vi "Cryotel Status.vi"(8 "Number of reads":i32, 11 "VISA Resource (write)":refnum<visa-resource-name>="COM1") -> (0 "Array 2":dbl[](array[numeric]), 3 "read string array":string[](array[string]))   [LabVIEW 2020]
uses:
  <vilib>/Analysis/baseanly.llb/Mean (DBL).vi
  <vilib>/Analysis/NI_AALBase.lvlib
panel:
  out "Array":string[](array[string])
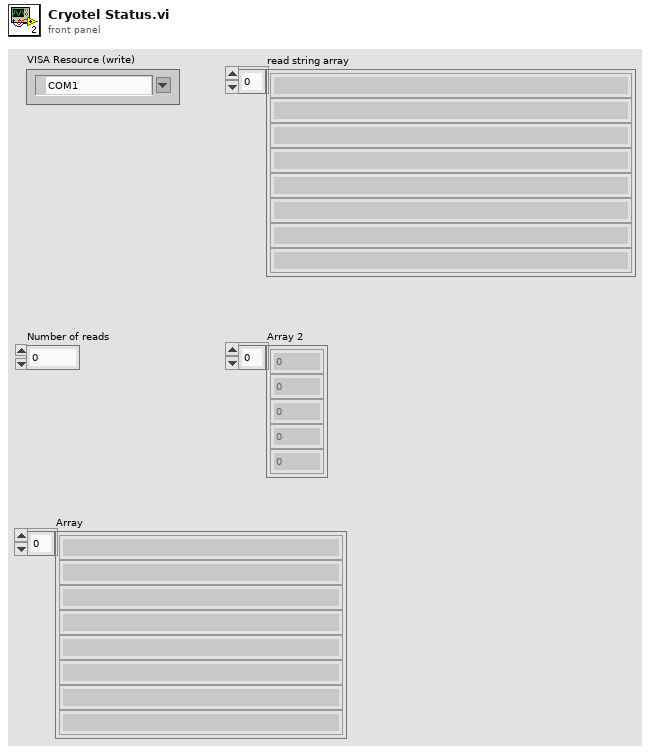
[diagram p1: front panel]
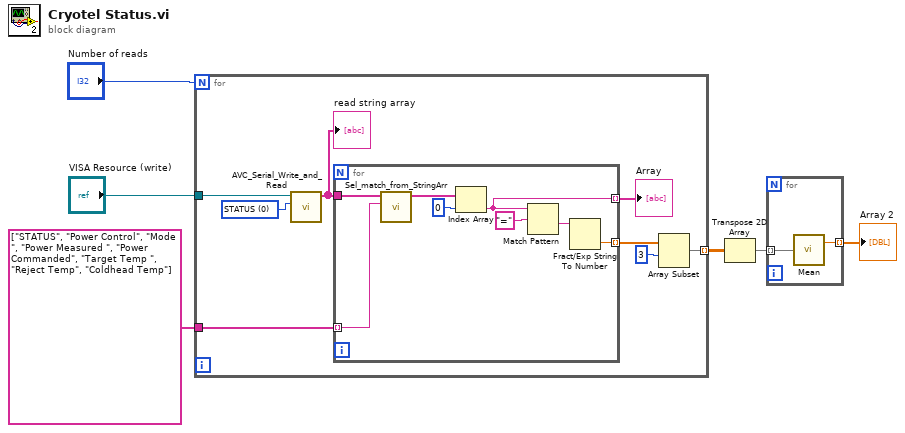
[diagram p0: block diagram]
diagram:
  n1 = for {
    N: "Number of reads" -> [_]
    tunnel: [w11] -> w2 mode=indexing
    tunnel: string[] ["STATUS", "Power Control", "Mode  ", "Power Measured ", "Power Commanded", "Target Temp ", "Reject Temp", "Coldhead Temp"] -> [w9]
    tunnel: "VISA Resource (write)" -> [w8]
    w7 = u16 0 items=["STATUS", "COOLER", "E", "ERROR", "KD", "KI", "KP", "LOGIN", "LOGOUT", "MODE", "P", "PWOUT", "SENSOR", "TC", "TEMP RJ", "TTARGET", "VERSION"] ("Command")
    n2 = call "AVC_Serial_Write_and_Read.vi"("Command"=w7, "VISA Resource (write)"=w8) -> ("read string array"=w10:string[])  [unwired: 8 in, 1 out]
    "read string array" <- w10
    n3 = for {
      tunnel: w10 -> [w22]
      tunnel: [w18] -> w14 mode=indexing
      tunnel: [w19] -> w12 mode=indexing
      tunnel: w9 -> [w15] mode=indexing
      n4 = call "Sel_match_from_StringArr.vi"("String to match"=w15, "String Array In"=w22) -> ("String Array Matched"=w21:string[])  [unwired: 6 in, 3 out]
      n5 = Index Array(array=w21, index=0) -> (element=w18:string)
      n6 = Match Pattern(string=w18, regular expression="=") -> (after substring=w16:string)  [unwired: 1 in, 3 out]
      n7 = Fract/Exp String To Number(string=w16) -> (number=w19:dbl)  [unwired: 3 in, 1 out]
    }
    "Array" <- w14
    n8 = Array Subset(array=w12, index=3) -> (w11:dbl[])  [unwired: 1 in]
  }
  n9 = Transpose 2D Array(2D array=w2) -> (transposed array=w3:dbl[][])
  n10 = for {
    tunnel: w3 -> [w24] mode=indexing
    tunnel: [w23] -> w1 mode=indexing
    n11 = call-poly <vilib>:"Mean.vi"("X"=w24) -> ("mean"=w23:dbl)  [unwired: 1 out]
  }
  "Array 2" <- w1
